vi "Fitting test.vi"() -> ()   [LabVIEW 2013]
panel:
  out "数组 4":dbl[][](array[numeric])
  out "sigy":i32
  out "yc":dbl
  out "sigx":i32
  out "xc":dbl
  out "peak":dbl
  in  "fitting type":dbl
  in  "force guess?":bool
  in  "noise3":dbl
  in  "数组 3":dbl[](array[numeric])
  in  "数组 2":dbl[](array[numeric])
  in  "数组":dbl[](array[numeric])
  in  "noise2":dbl
  out "x-y":u32
  out "best fit parameters":dbl[](array[numeric])
  out "强度图":dbl[][](graph)
  in  "noise":dbl
  in  "y":i32
  in  "x":i32
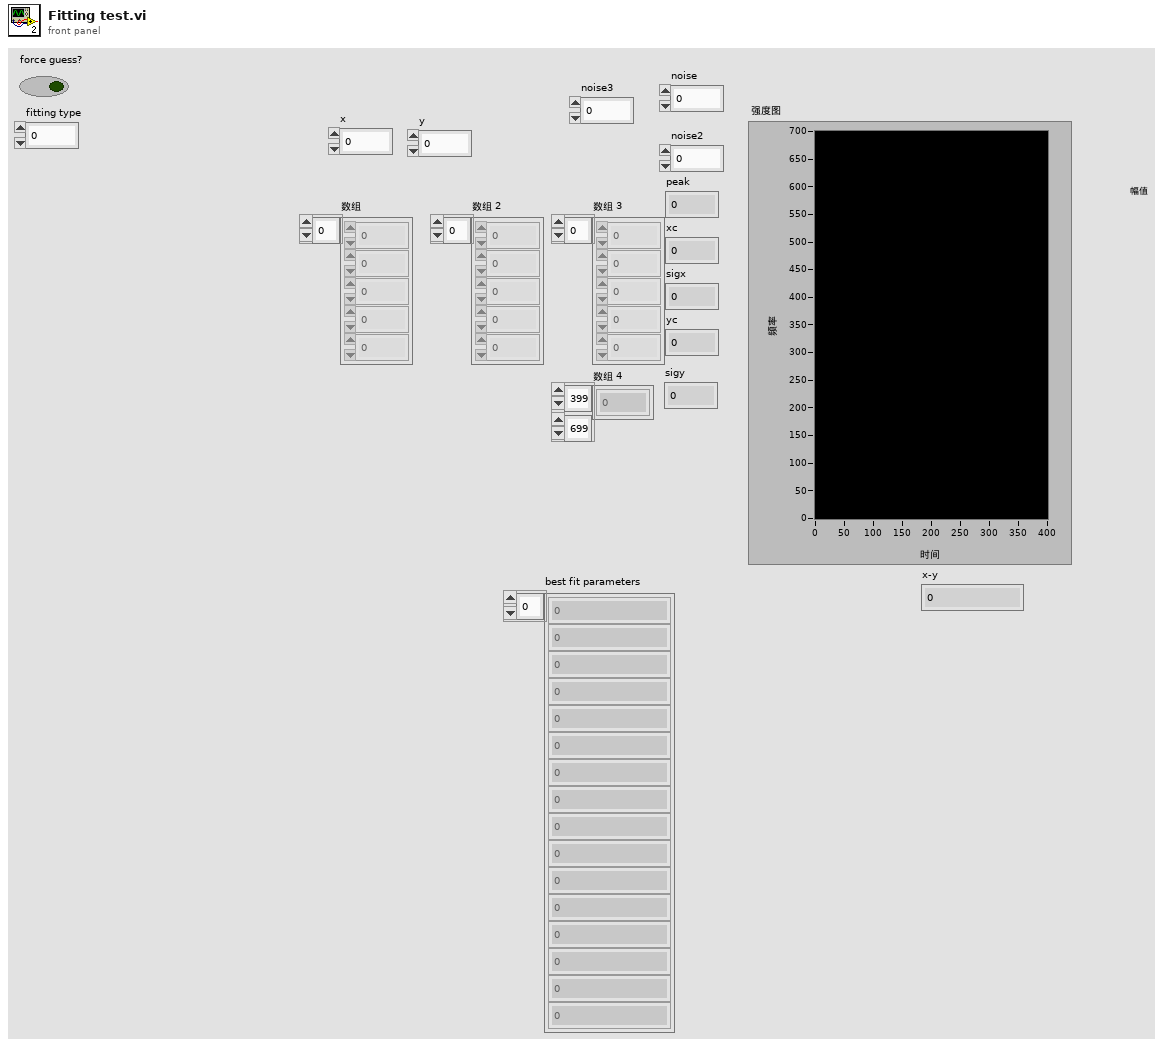
[diagram p1: front panel]
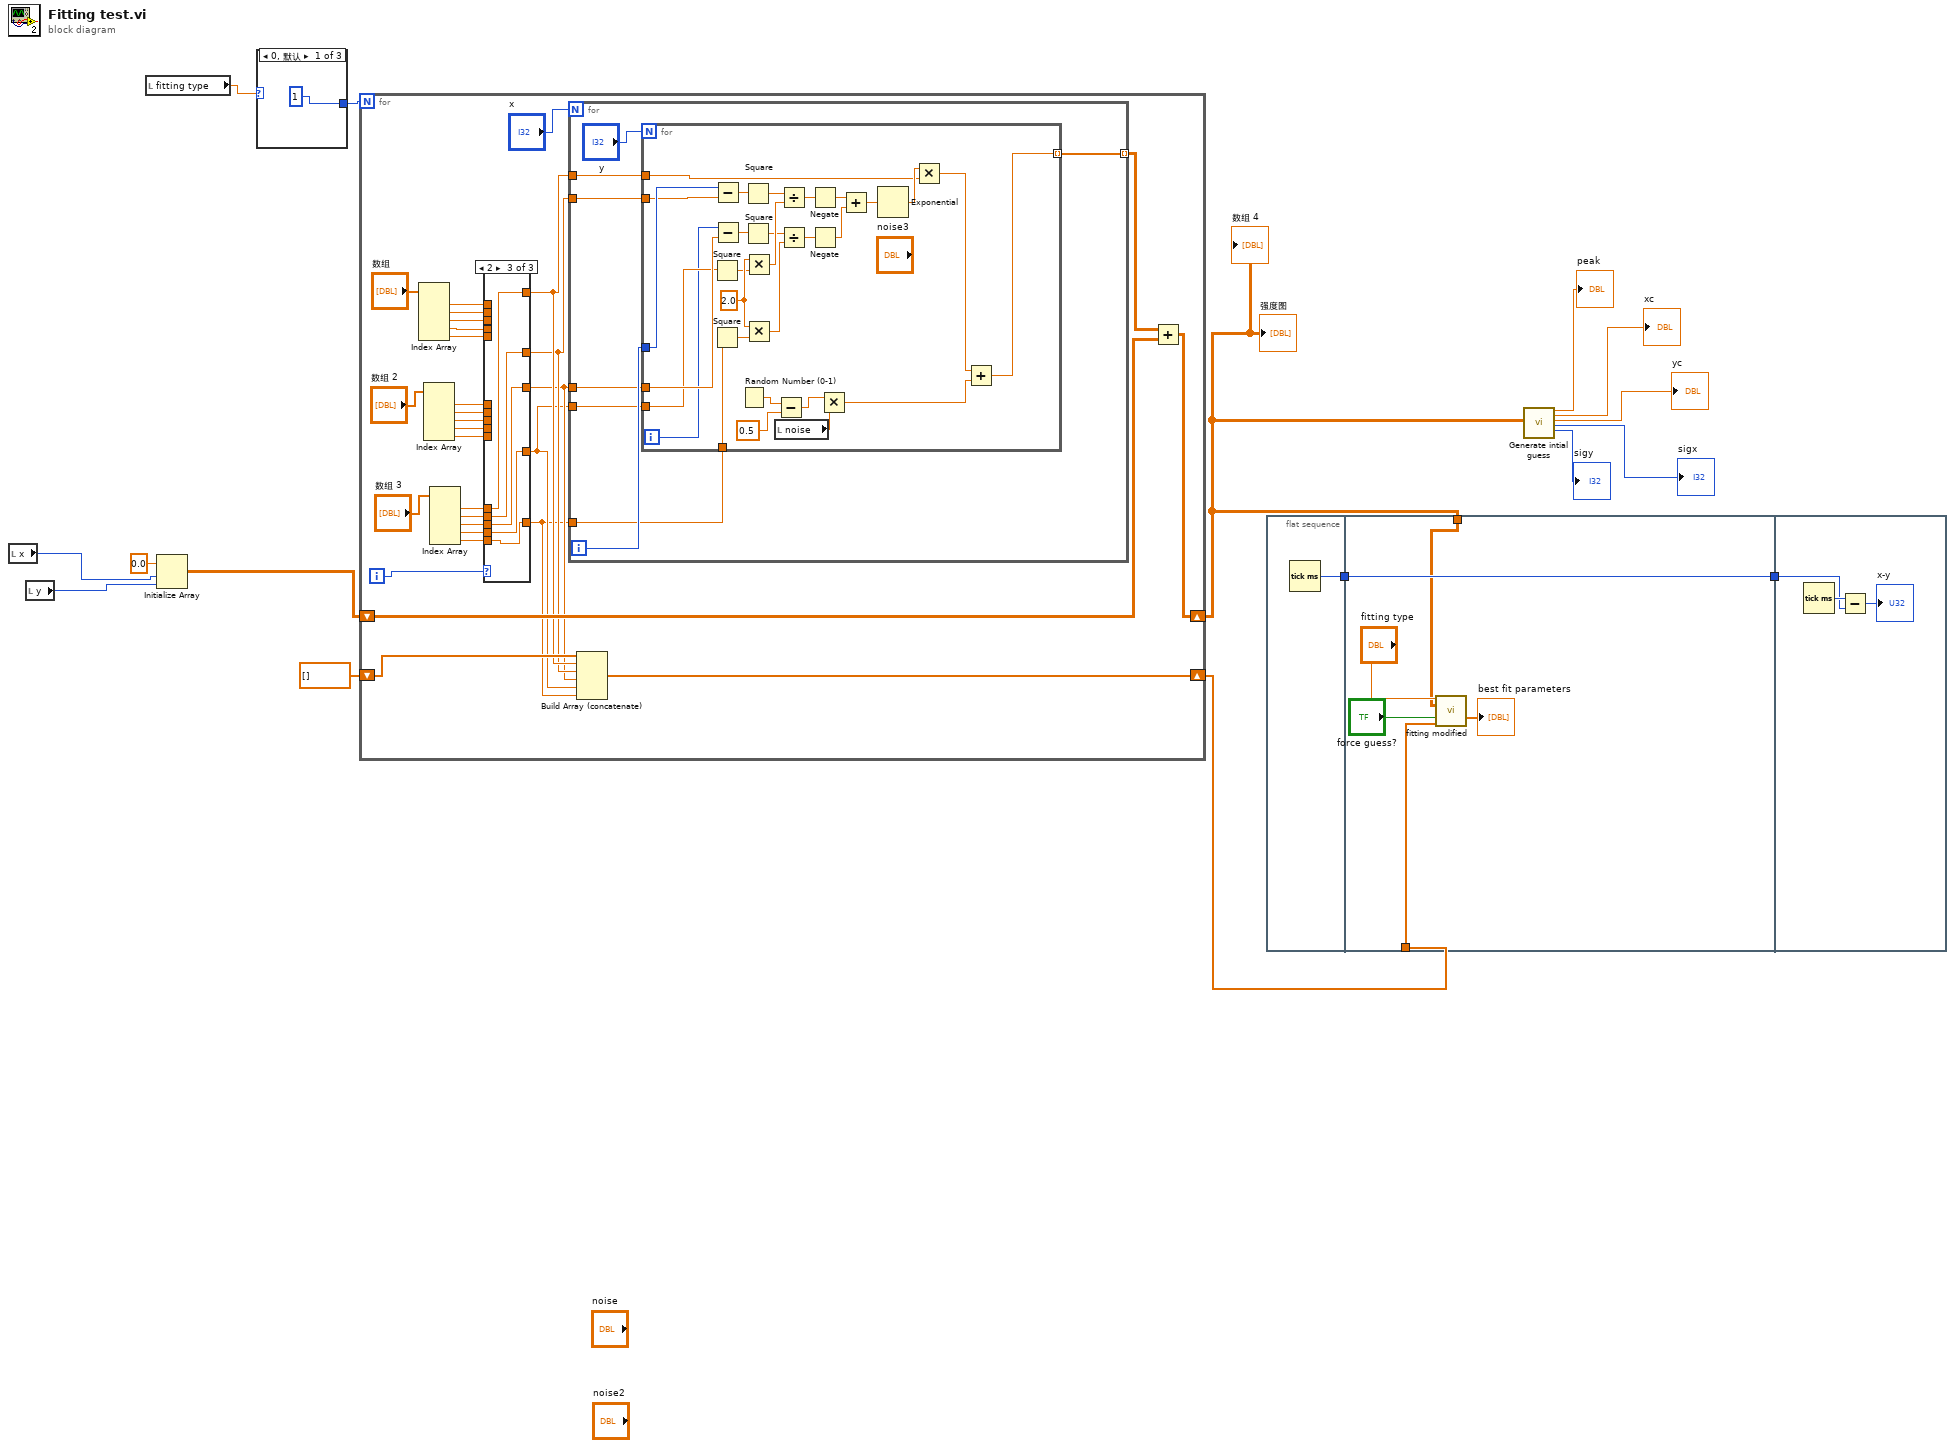
[diagram p0: block diagram]
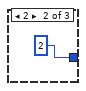
[diagram p2: hidden frame]
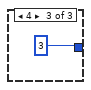
[diagram p3: hidden frame]
diagram:
  n1 = local read "x"() -> (w9:i32)
  n2 = local read "y"() -> (w8:i32)
  n3 = local read "fitting type"() -> (w14:dbl)
  n4 = Initialize Array(0.0 ("元素"), w9, w8) -> (w7:dbl[][])
  n5 = case shown="0, 默认" w14 {
    tunnel: [1 2 3] -> w13
    frame 0, Default {
    }
    frame 2 {
    }
    frame 4 {
    }
  }
  n6 = for {
    N: w13 -> [_]
    shift-right: [w28] -> w6
    shift-left: w7 -> [w27]
    shift-right: [w26] -> w11
    shift-left: dbl[] [] -> [w25]
    i -> [w45]
    n7 = Index Array(array="数组") -> (element #1=w44:dbl, element #2=w43:dbl, element #3=w42:dbl, element #4=w41:dbl, element #5=w40:dbl)  [unwired: 5 in]
    n8 = Index Array(array="数组 2") -> (element #1=w39:dbl, element #2=w38:dbl, element #3=w37:dbl, element #4=w36:dbl, element #5=w35:dbl)  [unwired: 5 in]
    n9 = Index Array(array="数组 3") -> (element #1=w34:dbl, element #2=w33:dbl, element #3=w32:dbl, element #4=w31:dbl, element #5=w30:dbl)  [unwired: 5 in]
    n10 = case shown="2" w45 {
      tunnel: w44 -> [w54 _ _]
      tunnel: w43 -> [w53 _ _]
      tunnel: w42 -> [w52 _ _]
      tunnel: w41 -> [w51 _ _]
      tunnel: w40 -> [w50 _ _]
      tunnel: w39 -> [_ w59 _]
      tunnel: w38 -> [_ w58 _]
      tunnel: w37 -> [_ w57 _]
      tunnel: w36 -> [_ w56 _]
      tunnel: w35 -> [_ w55 _]
      tunnel: w34 -> [_ _ w64]
      tunnel: w33 -> [_ _ w63]
      tunnel: w32 -> [_ _ w62]
      tunnel: w31 -> [_ _ w61]
      tunnel: w30 -> [_ _ w60]
      tunnel: [w54 w59 w64] -> w24
      tunnel: [w53 w58 w63] -> w23
      tunnel: [w52 w57 w62] -> w22
      tunnel: [w51 w56 w61] -> w21
      tunnel: [w50 w55 w60] -> w20
      frame 0, Default {
      }
      frame 1 {
      }
      frame 2 {
      }
    }
    n11 = for {
      N: "x" -> [_]
      tunnel: [w70] -> w29 mode=indexing
      tunnel: w24 -> [w69]
      tunnel: w23 -> [w68]
      tunnel: w22 -> [w67]
      tunnel: w21 -> [w66]
      tunnel: w20 -> [w65]
      i -> [w71]
      n12 = for {
        N: "y" -> [_]
        tunnel: w71 -> [w79]
        tunnel: [w81] -> w70 mode=indexing
        tunnel: w69 -> [w80]
        tunnel: w68 -> [w78]
        tunnel: w67 -> [w77]
        tunnel: w66 -> [w76]
        tunnel: w65 -> [w75]
        i -> [w74]
        w99 = 2.0 ("x")
        n13 = Square(x=w76) -> (x^2=w98:dbl)
        n14 = Square(x=w75) -> (x^2=w97:dbl)
        n15 = Subtract(x=w79, y=w78) -> (x-y=w101:dbl)
        n16 = Subtract(x=w74, y=w77) -> (x-y=w100:dbl)
        n17 = Random Number (0-1)() -> (number: 0 to 1=w86:dbl)
        n18 = Square(x=w101) -> (x^2=w96:dbl)
        n19 = Square(x=w100) -> (x^2=w94:dbl)
        n20 = Multiply(x=w99, y=w98) -> (x*y=w95:dbl)
        n21 = Multiply(x=w99, y=w97) -> (x*y=w93:dbl)
        n22 = local read "noise"() -> (w83:dbl)
        n23 = Subtract(x=w86, y=0.5) -> (x-y=w84:dbl)
        n24 = Divide(x=w96, y=w95) -> (x/y=w92:dbl)
        n25 = Divide(x=w94, y=w93) -> (x/y=w91:dbl)
        n26 = Negate(x=w92) -> (-x=w90:dbl)
        n27 = Negate(x=w91) -> (-x=w89:dbl)
        n28 = Multiply(x=w84, y=w83) -> (x*y=w82:dbl)
        n29 = Add(x=w90, y=w89) -> (x+y=w88:dbl)
        n30 = Exponential(1:w88) -> (0:w87:dbl)
        n31 = Multiply(x=w87, y=w80) -> (x*y=w73:dbl)
        n32 = Add(x=w73, y=w82) -> (x+y=w81:dbl)
      }
    }
    n33 = Build Array (concatenate)(w25, w24, w23, w22, w21, w20) -> (w26:dbl[])
    n34 = Add(x=w29, y=w27) -> (x+y=w28:dbl[][])
  }
  "强度图" <- w6
  "数组 4" <- w6
  n35 = flat-sequence {
    tunnel: [w102] -> w15
    tunnel: [w108] -> w16
    tunnel: w15 -> [w108]
    tunnel: w11 -> [w104]
    tunnel: w6 -> [w106]
    tunnel: w16 -> [w110]
    frame #0 {
      n36 = Tick Count (ms)() -> (millisecond timer value=w102:u32)
    }
    frame #1 {
      n37 = call "fitting modified.vi"("fitting type"="fitting type", "2D data"=w106, "force guess?"="force guess?", "intial guess value"=w104) -> ("best fit parameters"=→"best fit parameters":dbl[])  [unwired: 9 in, 2 out]
    }
    frame #2 {
      n38 = Tick Count (ms)() -> (millisecond timer value=w111:u32)
      n39 = Subtract(x=w111, y=w110) -> (x-y=→"x-y":u32)
    }
  }
  n40 = call "Generate intial guess.vi"("数组"=w6) -> ("peak"=→"peak":dbl, "xc"=→"xc":dbl, "yc"=→"yc":dbl, "sigx"=→"sigx":i32, "sigy"=→"sigy":i32)  [unwired: 14 in]
